vi "PH_AWG-510.Evt Call Read Settings.vi"(0 "i ref in":refnum<vi>, 1 "Instance":string, 2 "Pattern File":path, 5 "error in":errorcluster) -> (14 "i ref out":refnum<vi>, 19 "error out":errorcluster)   [LabVIEW 2014, in "PH_AWG-510.lvlib"]
doc: "This VI calls a method by a simple call."
uses:
  CSCore/CSSystem/CoreLib/CoreLib.string 2 byte array.vi
  PH_AWG-510.lvlib
  CSCore/CSSystem/CoreLib/CoreLib.lvlib
  CSCore/BaseProcess/BaseProcess.lvlib
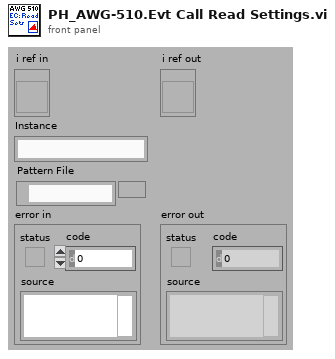
[diagram p1: front panel]
types:
  T1 = typedef "CoreDefs.rawDataType.ctl" = i8[]
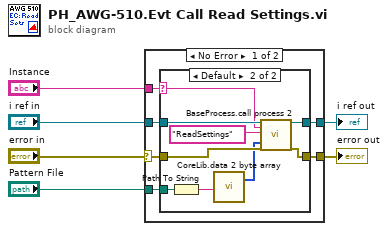
[diagram p0: block diagram]
diagram:
  n1 = case shown="No Error" "error in" {
    selector: "error in" -> [w8 w24]
    tunnel: [w12 w24] -> w3
    tunnel: "Instance" -> [w7 _]
    tunnel: "i ref in" -> [w11 w25]
    tunnel: [w10 w25] -> w5
    tunnel: "Pattern File" -> [w9 _]
    frame No Error {
      n2 = case shown="Default" w7 {
        selector: w7 -> [_ w17]
        tunnel: [w14 w23] -> w12
        tunnel: w8 -> [w14 w21]
        tunnel: w11 -> [w13 w20]
        tunnel: [w13 w19] -> w10
        tunnel: w9 -> [_ w18]
        frame "", "N/A" {
        }
        frame Default {
          n3 = Path To String(path=w18) -> (string=w16:string)
          n4 = call-poly "CoreLib.data 2 byte array.vi"("string"=w16) -> ("byteArray out"=w15:T1)  [unwired: 18 in]
          n5 = call "BaseProcess.call process 2.vi"("i ref in"=w20, "Object"=w17, "Selector"="ReadSettings", "Data"=w15, "error in (no error)"=w21) -> ("i ref out"=w19:refnum<vi>, "error out"=w23:errorcluster)  [unwired: 13 in]
        }
      }
    }
    frame Error {
    }
  }
  "i ref out" <- w5
  "error out" <- w3
